vi "Multiply Force.vi"(10 "force in":dbl, 11 "House Key in":refnum<class "House Key.lvclass">) -> (2 "force out":dbl)   [LabVIEW 2023, in "House Key.lvclass"]
uses:
  House Key.lvclass
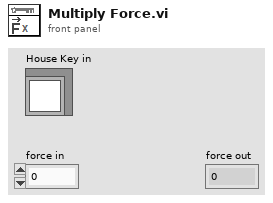
[diagram p1: front panel]
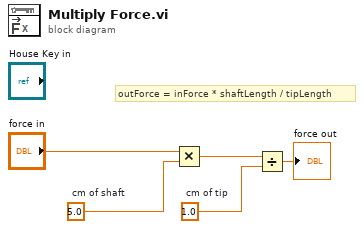
[diagram p0: block diagram]
diagram:
  w4 = 5.0  # cm of shaft
  w5 = 1.0  # cm of tip
  # "outForce = inForce * shaftLength / tipLength"
  n1 = Multiply(x="force in", y=w4) -> (x*y=w2:dbl)
  n2 = Divide(x=w2, y=w5) -> (x/y=→"force out":dbl)
